vi "Control AlgorithmV3.vi"(6 "PID Gains":cluster{"P":dbl, "I":dbl, "D":dbl}, 7 "Init":bool, 8 "Motor to Control":u8, 9 "Manual Control":bool, 10 "Wheel Angles":dbl[](array[numeric]), 11 "JoystickIn":i32[](array[slide]) scale=-37626.0..37626.0) -> (2 "Target Angles":dbl[](array[numeric]), 3 "MotorsOut":u16[](array[slide]) scale=0.0..512.0)   [LabVIEW 2013, in "ProcessorHelperFunctions.lvlib"]
uses:
  ProcessorHelperFunctions.lvlib
panel:
  out "JoystickIn_DB":i32[](array[slide]) scale=-37626.0..37626.0
  out "y":dbl
  out "x":dbl
  out "Point":picture
  out "ReverseDir?4":bool
  out "ReverseDir?3":bool
  out "ReverseDir?2":bool
  out "ReverseDir?1":bool
  out "Radius1":dbl
  out "Radius2":dbl
  out "Radius3":dbl
  out "Radius4":dbl
  in  "RJoyMagGain":dbl=0.25
  in  "LJoyMagGain":dbl=1.0
  out "OldAngle4":dbl
  out "OldAngle3":dbl
  out "OldAngle2":dbl
  out "OldAngle1":dbl
  in  "Yw":dbl=15.5
  in  "Xw":dbl=21.5
  # "Xw is x distance between the\nwheels on the robot"
  # "------------------------------------ LOCAL VARIABLES ---------------------------------------"
  # "Yw is y distance between the\nwheels on the robot"
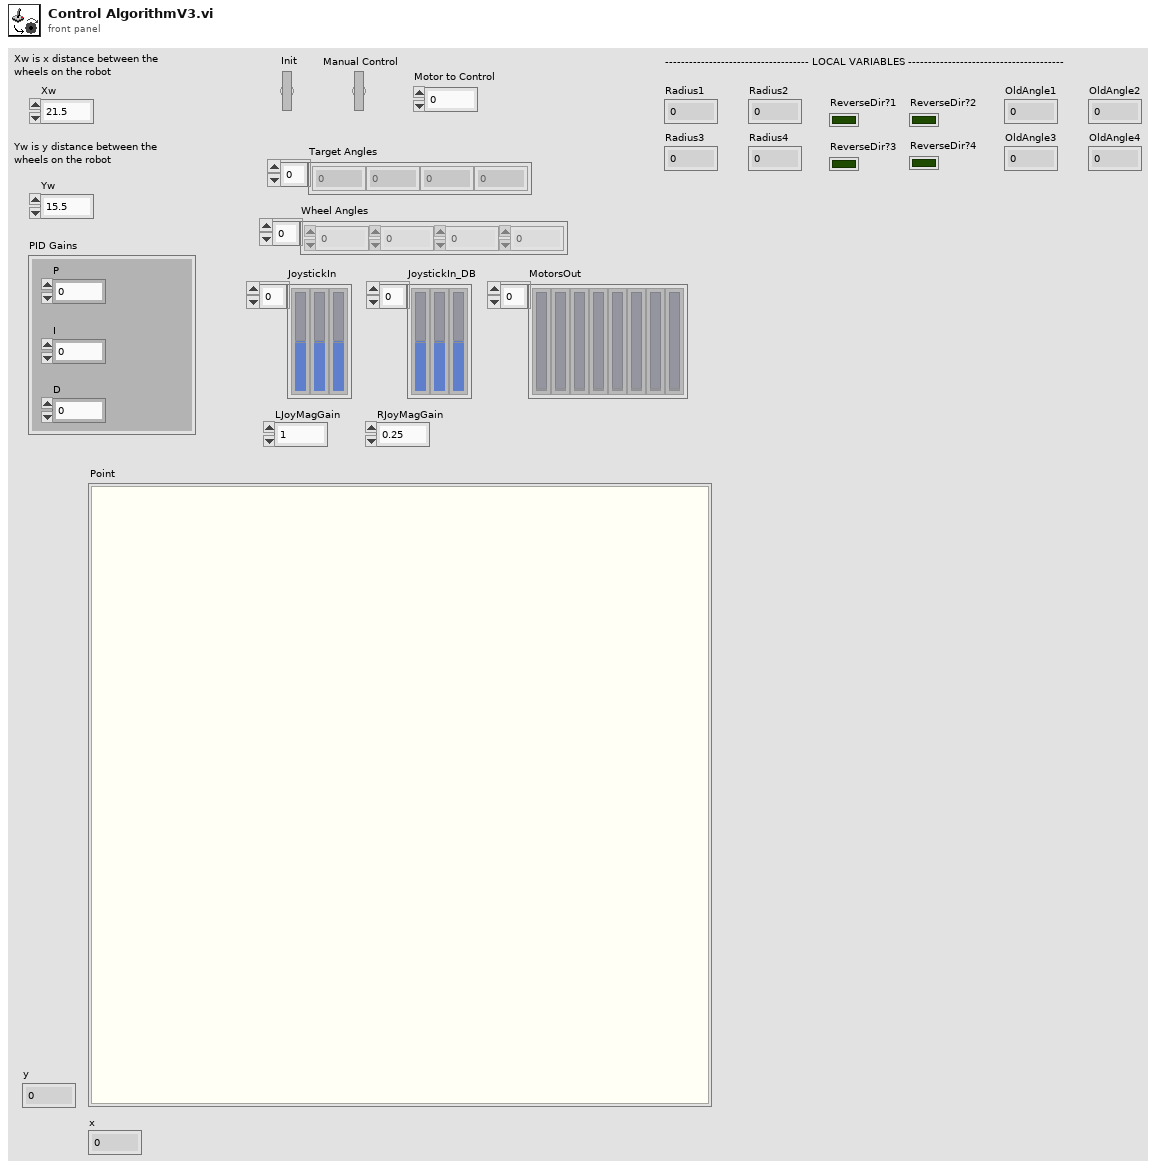
[diagram p1: front panel]
types:
  T1 = cluster{"Width":u16, "Style":enum32{"Solid", "Dash", "Dot", "DashDot", "DashDotDot"}}
  T2 = cluster{"JoystickOut[0]":i32, "JoystickOut[1]":i32, "JoystickOut[2]":i32, "JoystickOut[3]":i32, "JoystickOut[4]":i32, "JoystickOut[5]":i32, "JoystickOut[6]":i32, "JoystickOut[7]":i32, "JoystickOut[8]":i32}
  T3 = cluster{"Wheel Angles[0]":dbl, "Wheel Angles[1]":dbl, "Wheel Angles[2]":dbl, "Wheel Angles[3]":dbl, "Wheel Angles[4]":dbl, "Wheel Angles[5]":dbl, "Wheel Angles[6]":dbl, "Wheel Angles[7]":dbl, "Wheel Angles[8]":dbl}
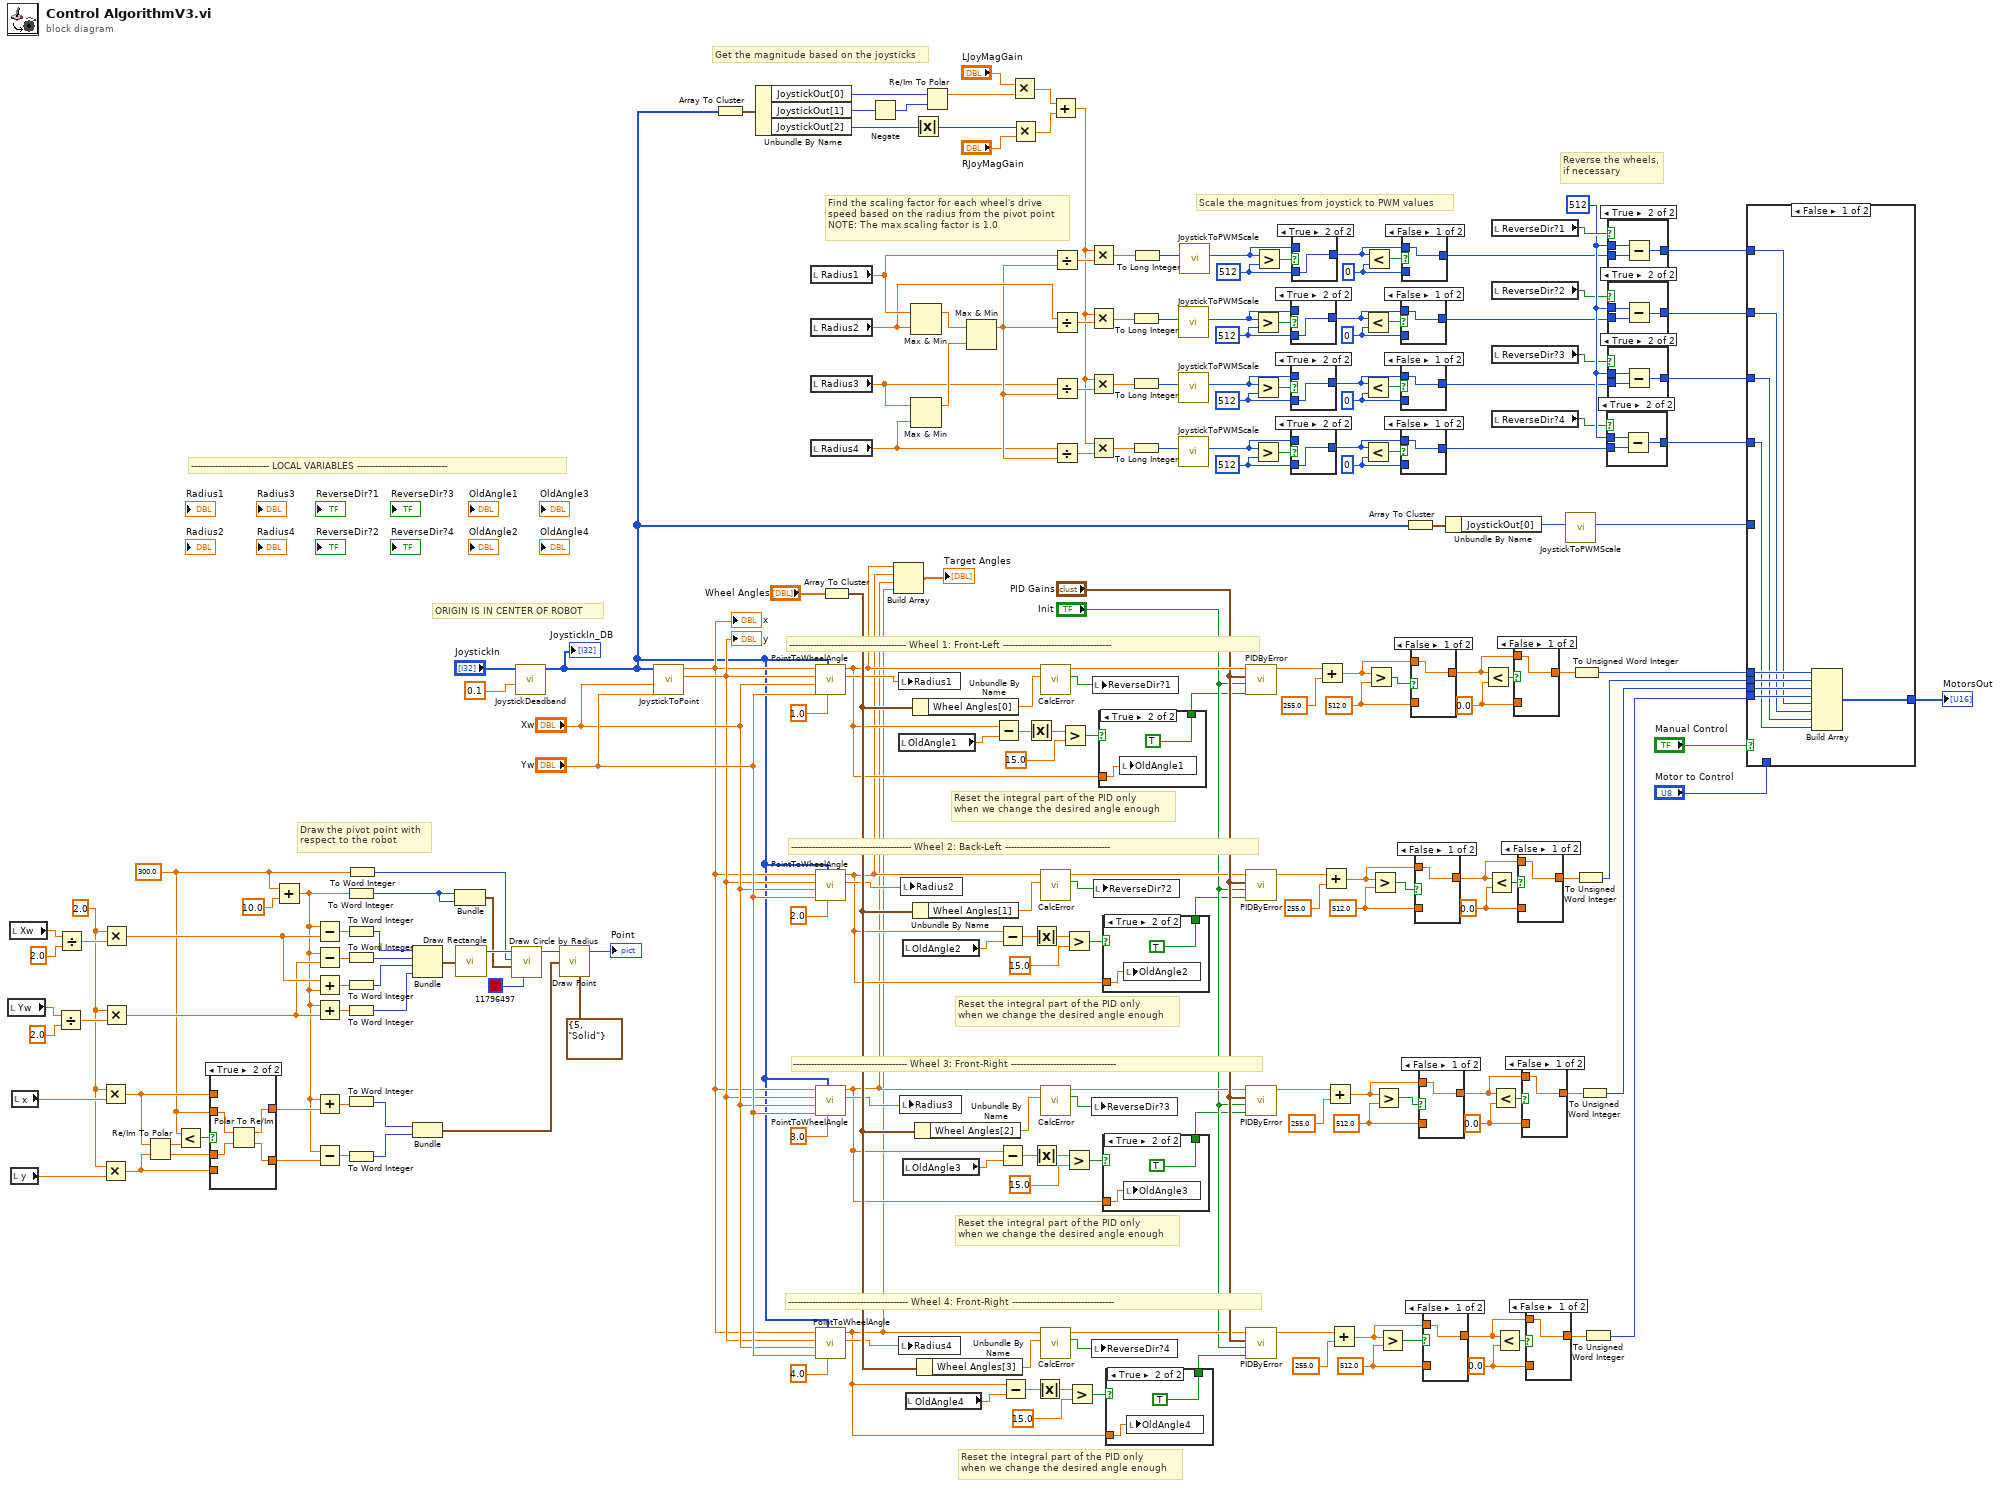
[diagram p0: block diagram]
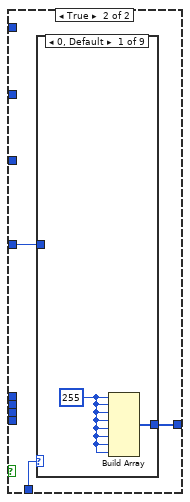
[diagram p15: hidden frame]
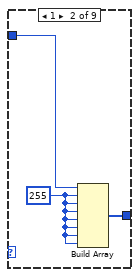
[diagram p16: hidden frame]
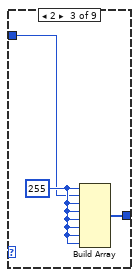
[diagram p17: hidden frame]
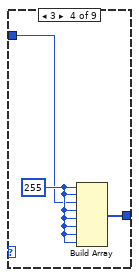
[diagram p18: hidden frame]
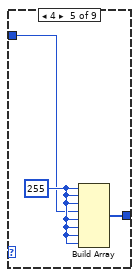
[diagram p19: hidden frame]
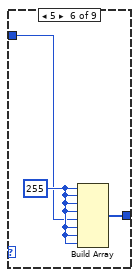
[diagram p20: hidden frame]
diagram:
  w7 = 0 ("y")
  w8 = 512 ("y")
  w18 = 0 ("y")
  w17 = 512 ("y")
  w25 = 0 ("y")
  w26 = 512 ("y")
  w41 = u16 512 ("x")
  w72 = 2.0 ("x")
  w53 = 300.0 ("x")
  w123 = 0 ("y")
  w122 = 512 ("y")
  w147 = 0.0 ("y")
  w145 = 512.0 ("y")
  w153 = 0.0 ("y")
  w155 = 512.0 ("y")
  w163 = 0.0 ("y")
  w161 = 512.0 ("y")
  w168 = 0.0 ("y")
  w170 = 512.0 ("y")
  # "Scale the magnitues from joystick to PWM values"
  # "Get the magnitude based on the joysticks"
  # "Reverse the wheels,\nif necessary"
  # "Draw the pivot point with\nrespect to the robot"
  # "Find the scaling factor for each wheel's drive\nspeed based on the radius from the pivot point\nNOTE: The max scaling factor is 1.0"
  # "Reset the integral part of the PID only\nwhen we change the desired angle enough"
  # "Reset the integral part of the PID only\nwhen we change the desired angle enough"
  # "Reset the integral part of the PID only\nwhen we change the desired angle enough"
  # "Reset the integral part of the PID only\nwhen we change the desired angle enough"
  # "-------------------------- LOCAL VARIABLES ------------------------------"
  # "---------------------------------------- Wheel 4: Front-Right ----------------------------------"
  # "-------------------------------------- Wheel 3: Front-Right -----------------------------------"
  # "---------------------------------------- Wheel 2: Back-Left -----------------------------------"
  # "--------------------------------------- Wheel 1: Front-Left ------------------------------------"
  # "ORIGIN IS IN CENTER OF ROBOT"
  n1 = local read "Yw"() -> (w97:dbl)
  n2 = local read "Xw"() -> (w100:dbl)
  n3 = local read "y"() -> (w73:dbl)
  n4 = local read "x"() -> (w80:dbl)
  n5 = Divide(x=w97, y=2.0) -> (x/y=w77:dbl)
  n6 = Divide(x=w100, y=2.0) -> (x/y=w78:dbl)
  n7 = Multiply(x=w72, y=w80) -> (x*y=w67:dbl)
  n8 = Multiply(x=w72, y=w73) -> (x*y=w66:dbl)
  n9 = Multiply(x=w72, y=w78) -> (x*y=w75:dbl)
  n10 = Multiply(x=w72, y=w77) -> (x*y=w74:dbl)
  n11 = Re/Im To Polar(2:w66, 3:w67) -> (0:w65:dbl, 1:w69:dbl)
  n12 = Less?(x=w53, y=w69) -> (x < y?=w68:bool)
  n13 = case shown="True" w68 {
    tunnel: w67 -> [w219 _]
    tunnel: w66 -> [w218 _]
    tunnel: w53 -> [_ w223]
    tunnel: w65 -> [_ w222]
    tunnel: [w219 w221] -> w63
    tunnel: [w218 w220] -> w64
    frame False {
    }
    frame True {
      n14 = Polar To Re/Im(2:w222, 3:w223) -> (0:w220:dbl, 1:w221:dbl)
    }
  }
  n15 = Add(x=w53, y=10.0) -> (x+y=w52:dbl)
  n16 = Subtract(x=w52, y=w75) -> (x-y=w58:dbl)
  n17 = Subtract(x=w52, y=w74) -> (x-y=w87:dbl)
  n18 = Add(x=w75, y=w52) -> (x+y=w86:dbl)
  n19 = Add(x=w52, y=w74) -> (x+y=w85:dbl)
  n20 = Add(x=w52, y=w63) -> (x+y=w62:dbl)
  n21 = Subtract(x=w52, y=w64) -> (x-y=w61:dbl)
  n22 = To Word Integer(number=w52) -> (16bit integer=w51:i16)
  n23 = To Word Integer(number=w58) -> (16bit integer=w88:i16)
  n24 = To Word Integer(number=w87) -> (16bit integer=w84:i16)
  n25 = To Word Integer(number=w86) -> (16bit integer=w83:i16)
  n26 = To Word Integer(number=w85) -> (16bit integer=w82:i16)
  n27 = To Word Integer(number=w62) -> (16bit integer=w96:i16)
  n28 = To Word Integer(number=w61) -> (16bit integer=w95:i16)
  n29 = To Word Integer(number=w53) -> (16bit integer=w55:i16)
  n30 = Bundle(w88, w84, w83, w82) -> (w81:cluster{i16, i16, i16, i16})  [unwired: 1 in]
  n31 = Bundle(w96, w95) -> (w94:cluster{i16, i16})  [unwired: 1 in]
  n32 = Bundle(w51, w51) -> (w57:cluster{i16, i16})  [unwired: 1 in]
  n33 = call <vilib>:"Draw Rectangle.vi"("rect"=w81) -> ("new picture"=w60:picture)  [unwired: 8 in]
  n34 = call <vilib>:"Draw Circle by Radius.vi"("color(black)"=u32 11796497, "pixel center"=w57, "radius"=w55, "picture"=w60) -> ("new picture"=w59:picture)  [unwired: 7 in]
  n35 = call "JoystickDeadband.vi"("DBPercent"=0.1, "JoystickIn"="JoystickIn") -> ("JoystickOut"=w2:i32[])  [unwired: 9 in]
  "JoystickIn_DB" <- w2
  n36 = call <vilib>:"Draw Point.vi"("picture"=w59, "point(x,y)"=w94, "pen"=T1 {"Width"=5, "Style"=enum."Solid"}) -> ("new picture"=→"Point":picture)  [unwired: 6 in]
  n37 = call "JoystickToPoint.vi"("Yw"="Yw", "Xw"="Xw", "JoystickIn"=w2) -> ("y"=w211:dbl, "x"=w210:dbl)  [unwired: 7 in]
  "x" <- w210
  "y" <- w211
  n38 = Array To Cluster(array=w2) -> (cluster=w134:T2)
  n39 = Unbundle By Name(w134) -> ("JoystickOut[0]"=w133:i32, "JoystickOut[1]"=w132:i32, "JoystickOut[2]"=w129:i32)
  n40 = local read "Radius1"() -> (w109:dbl)
  n41 = local read "Radius2"() -> (w108:dbl)
  n42 = local read "Radius3"() -> (w106:dbl)
  n43 = local read "Radius4"() -> (w105:dbl)
  n44 = call "PointToWheelAngle.vi"("Wheel Number"=1.0, "JoystickIn"=w2, "Yw"="Yw", "Xw"="Xw", "y"=w211, "x"=w210) -> ("Radius"=w119:dbl, "Desired Angle"=w50:dbl)  [unwired: 4 in]
  n45 = call "PointToWheelAngle.vi"("Wheel Number"=2.0, "JoystickIn"=w2, "Yw"="Yw", "Xw"="Xw", "y"=w211, "x"=w210) -> ("Radius"=w118:dbl, "Desired Angle"=w49:dbl)  [unwired: 4 in]
  n46 = call "PointToWheelAngle.vi"("Wheel Number"=3.0, "JoystickIn"=w2, "Yw"="Yw", "Xw"="Xw", "y"=w211, "x"=w210) -> ("Radius"=w117:dbl, "Desired Angle"=w48:dbl)  [unwired: 4 in]
  n47 = call "PointToWheelAngle.vi"("Wheel Number"=4.0, "JoystickIn"=w2, "Yw"="Yw", "Xw"="Xw", "y"=w211, "x"=w210) -> ("Radius"=w116:dbl, "Desired Angle"=w47:dbl)  [unwired: 4 in]
  n48 = Array To Cluster(array="Wheel Angles") -> (cluster=w208:T3)
  n49 = Negate(x=w132) -> (-x=w76:i32)
  n50 = Build Array(w50, w49, w48, w47) -> (→"Target Angles":dbl[])
  n51 = local write "Radius1"(w119) -> ()
  n52 = local read "OldAngle1"() -> (w198:dbl)
  n53 = local write "Radius4"(w116) -> ()
  n54 = local write "Radius3"(w117) -> ()
  n55 = local write "Radius2"(w118) -> ()
  n56 = local read "OldAngle2"() -> (w191:dbl)
  n57 = local read "OldAngle3"() -> (w186:dbl)
  n58 = local read "OldAngle4"() -> (w181:dbl)
  n59 = Max & Min(x=w109, y=w108) -> (max(x,y)=w111:dbl)  [unwired: 1 out]
  n60 = Max & Min(x=w106, y=w105) -> (max(x,y)=w110:dbl)  [unwired: 1 out]
  n61 = Absolute Value(x=w129) -> (abs(x)=w1:i32)
  n62 = Unbundle By Name(w208) -> ("Wheel Angles[0]"=w207:dbl)
  n63 = Unbundle By Name(w208) -> ("Wheel Angles[1]"=w206:dbl)
  n64 = Unbundle By Name(w208) -> ("Wheel Angles[2]"=w205:dbl)
  n65 = Unbundle By Name(w208) -> ("Wheel Angles[3]"=w204:dbl)
  n66 = Re/Im To Polar(2:w76, 3:w133) -> (1:w131:dbl)  [unwired: 1 out]
  n67 = Max & Min(x=w111, y=w110) -> (max(x,y)=w107:dbl)  [unwired: 1 out]
  n68 = Subtract(x=w50, y=w198) -> (x-y=w197:dbl)
  n69 = Subtract(x=w49, y=w191) -> (x-y=w190:dbl)
  n70 = Subtract(x=w48, y=w186) -> (x-y=w185:dbl)
  n71 = Subtract(x=w47, y=w181) -> (x-y=w180:dbl)
  n72 = Multiply(x="LJoyMagGain", y=w131) -> (x*y=w127:dbl)
  n73 = Multiply(x=w1, y="RJoyMagGain") -> (x*y=w126:dbl)
  n74 = Absolute Value(x=w197) -> (abs(x)=w196:dbl)
  n75 = Absolute Value(x=w190) -> (abs(x)=w189:dbl)
  n76 = Absolute Value(x=w185) -> (abs(x)=w184:dbl)
  n77 = Absolute Value(x=w180) -> (abs(x)=w179:dbl)
  n78 = call "CalcError.vi"("Actual Angle"=w207, "Desired Angle"=w50) -> ("ReverseDir?"=w115:bool, "Angle Error"=w203:dbl)  [unwired: 8 in]
  n79 = call "CalcError.vi"("Actual Angle"=w206, "Desired Angle"=w49) -> ("ReverseDir?"=w114:bool, "Angle Error"=w201:dbl)  [unwired: 8 in]
  n80 = call "CalcError.vi"("Actual Angle"=w205, "Desired Angle"=w48) -> ("ReverseDir?"=w113:bool, "Angle Error"=w200:dbl)  [unwired: 8 in]
  n81 = call "CalcError.vi"("Actual Angle"=w204, "Desired Angle"=w47) -> ("ReverseDir?"=w112:bool, "Angle Error"=w199:dbl)  [unwired: 8 in]
  n82 = Add(x=w127, y=w126) -> (x+y=w32:dbl)
  n83 = Divide(x=w109, y=w107) -> (x/y=w36:dbl)
  n84 = Divide(x=w108, y=w107) -> (x/y=w35:dbl)
  n85 = Divide(x=w106, y=w107) -> (x/y=w34:dbl)
  n86 = Divide(x=w105, y=w107) -> (x/y=w33:dbl)
  n87 = Greater?(x=w196, y=15.0) -> (0:w194:bool)
  n88 = Greater?(x=w189, y=15.0) -> (0:w187:bool)
  n89 = Greater?(x=w184, y=15.0) -> (0:w182:bool)
  n90 = Greater?(x=w179, y=15.0) -> (0:w177:bool)
  n91 = Multiply(x=w32, y=w36) -> (x*y=w31:dbl)
  n92 = Multiply(x=w32, y=w35) -> (x*y=w22:dbl)
  n93 = Multiply(x=w32, y=w34) -> (x*y=w13:dbl)
  n94 = Multiply(x=w32, y=w33) -> (x*y=w4:dbl)
  n95 = local write "ReverseDir?3"(w113) -> ()
  n96 = local write "ReverseDir?4"(w112) -> ()
  n97 = local write "ReverseDir?1"(w115) -> ()
  n98 = local write "ReverseDir?2"(w114) -> ()
  n99 = case shown="True" w194 {
    tunnel: w50 -> [_ w226]
    tunnel: [FALSE ("Reset1") TRUE ("Reset1")] -> w192
    frame False {
    }
    frame True {
      n100 = local write "OldAngle1"(w226) -> ()
    }
  }
  n101 = case shown="True" w187 {
    tunnel: w49 -> [_ w229]
    tunnel: [FALSE ("Reset1") TRUE ("Reset1")] -> w174
    frame False {
    }
    frame True {
      n102 = local write "OldAngle2"(w229) -> ()
    }
  }
  n103 = case shown="True" w182 {
    tunnel: w48 -> [_ w232]
    tunnel: [FALSE ("Reset1") TRUE ("Reset1")] -> w176
    frame False {
    }
    frame True {
      n104 = local write "OldAngle3"(w232) -> ()
    }
  }
  n105 = case shown="True" w177 {
    tunnel: w47 -> [_ w235]
    tunnel: [FALSE ("Reset1") TRUE ("Reset1")] -> w175
    frame False {
    }
    frame True {
      n106 = local write "OldAngle4"(w235) -> ()
    }
  }
  n107 = To Long Integer(number=w22) -> (32bit integer=w23:i32)
  n108 = To Long Integer(number=w13) -> (32bit integer=w20:i32)
  n109 = To Long Integer(number=w4) -> (32bit integer=w5:i32)
  n110 = To Long Integer(number=w31) -> (32bit integer=w125:i32)
  n111 = call "JoystickToPWMScale.vi"("Numeric"=w23) -> ("Numeric 2"=w28:u16)  [unwired: 10 in]
  n112 = call "JoystickToPWMScale.vi"("Numeric"=w20) -> ("Numeric 2"=w15:u16)  [unwired: 10 in]
  n113 = call "JoystickToPWMScale.vi"("Numeric"=w5) -> ("Numeric 2"=w10:u16)  [unwired: 10 in]
  n114 = call "JoystickToPWMScale.vi"("Numeric"=w125) -> ("Numeric 2"=w120:u16)  [unwired: 10 in]
  n115 = call "PIDByError.vi"("Error"=w203, "PID Gains"="PID Gains", "Init"="Init", "Reset"=w192) -> ("Control"=w173:dbl)  [unwired: 6 in]
  n116 = call "PIDByError.vi"("Error"=w201, "PID Gains"="PID Gains", "Init"="Init", "Reset"=w174) -> ("Control"=w158:dbl)  [unwired: 6 in]
  n117 = call "PIDByError.vi"("Error"=w200, "PID Gains"="PID Gains", "Init"="Init", "Reset"=w176) -> ("Control"=w150:dbl)  [unwired: 6 in]
  n118 = call "PIDByError.vi"("Error"=w199, "PID Gains"="PID Gains", "Init"="Init", "Reset"=w175) -> ("Control"=w142:dbl)  [unwired: 6 in]
  n119 = Greater?(x=w28, y=w26) -> (0:w27:bool)
  n120 = Greater?(x=w15, y=w17) -> (0:w16:bool)
  n121 = Greater?(x=w10, y=w8) -> (0:w9:bool)
  n122 = Greater?(x=w120, y=w122) -> (0:w121:bool)
  n123 = case shown="True" w27 {
    tunnel: w26 -> [_ w237]
    tunnel: w28 -> [w236 _]
    tunnel: [w236 w237] -> w24
    frame False {
    }
    frame True {
    }
  }
  n124 = case shown="True" w16 {
    tunnel: w17 -> [_ w239]
    tunnel: w15 -> [w238 _]
    tunnel: [w238 w239] -> w19
    frame False {
    }
    frame True {
    }
  }
  n125 = case shown="True" w9 {
    tunnel: w8 -> [_ w241]
    tunnel: w10 -> [w240 _]
    tunnel: [w240 w241] -> w6
    frame False {
    }
    frame True {
    }
  }
  n126 = case shown="True" w121 {
    tunnel: w122 -> [_ w243]
    tunnel: w120 -> [w242 _]
    tunnel: [w242 w243] -> w124
    frame False {
    }
    frame True {
    }
  }
  n127 = Add(x=w173, y=255.0) -> (x+y=w169:dbl)
  n128 = Add(x=w158, y=255.0) -> (x+y=w162:dbl)
  n129 = Add(x=w150, y=255.0) -> (x+y=w154:dbl)
  n130 = Add(x=w142, y=255.0) -> (x+y=w146:dbl)
  n131 = Less?(x=w24, y=w25) -> (x < y?=w29:bool)
  n132 = Less?(x=w19, y=w18) -> (x < y?=w14:bool)
  n133 = Less?(x=w6, y=w7) -> (x < y?=w11:bool)
  n134 = Less?(x=w124, y=w123) -> (x < y?=w89:bool)
  n135 = Greater?(x=w169, y=w170) -> (0:w171:bool)
  n136 = Greater?(x=w162, y=w161) -> (0:w160:bool)
  n137 = Greater?(x=w154, y=w155) -> (0:w156:bool)
  n138 = Greater?(x=w146, y=w145) -> (0:w144:bool)
  n139 = case shown="False" w29 {
    tunnel: w25 -> [_ w245]
    tunnel: w24 -> [w244 _]
    tunnel: [w244 w245] -> w21
    frame False {
    }
    frame True {
    }
  }
  n140 = case shown="False" w14 {
    tunnel: w18 -> [_ w247]
    tunnel: w19 -> [w246 _]
    tunnel: [w246 w247] -> w12
    frame False {
    }
    frame True {
    }
  }
  n141 = case shown="False" w11 {
    tunnel: w7 -> [_ w249]
    tunnel: w6 -> [w248 _]
    tunnel: [w248 w249] -> w3
    frame False {
    }
    frame True {
    }
  }
  n142 = case shown="False" w89 {
    tunnel: w123 -> [_ w251]
    tunnel: w124 -> [w250 _]
    tunnel: [w250 w251] -> w30
    frame False {
    }
    frame True {
    }
  }
  n143 = Array To Cluster(array=w2) -> (cluster=w104:T2)
  n144 = case shown="False" w171 {
    tunnel: w170 -> [_ w253]
    tunnel: w169 -> [w252 _]
    tunnel: [w252 w253] -> w167
    frame False {
    }
    frame True {
    }
  }
  n145 = case shown="False" w160 {
    tunnel: w161 -> [_ w255]
    tunnel: w162 -> [w254 _]
    tunnel: [w254 w255] -> w164
    frame False {
    }
    frame True {
    }
  }
  n146 = case shown="False" w156 {
    tunnel: w155 -> [_ w257]
    tunnel: w154 -> [w256 _]
    tunnel: [w256 w257] -> w152
    frame False {
    }
    frame True {
    }
  }
  n147 = case shown="False" w144 {
    tunnel: w145 -> [_ w259]
    tunnel: w146 -> [w258 _]
    tunnel: [w258 w259] -> w148
    frame False {
    }
    frame True {
    }
  }
  n148 = Unbundle By Name(w104) -> ("JoystickOut[0]"=w103:i32)
  n149 = Less?(x=w167, y=w168) -> (x < y?=w90:bool)
  n150 = Less?(x=w164, y=w163) -> (x < y?=w91:bool)
  n151 = Less?(x=w152, y=w153) -> (x < y?=w92:bool)
  n152 = local read "ReverseDir?1"() -> (w45:bool)
  n153 = local read "ReverseDir?2"() -> (w39:bool)
  n154 = local read "ReverseDir?3"() -> (w38:bool)
  n155 = local read "ReverseDir?4"() -> (w37:bool)
  n156 = Less?(x=w148, y=w147) -> (x < y?=w93:bool)
  n157 = case shown="False" w90 {
    tunnel: w168 -> [_ w261]
    tunnel: w167 -> [w260 _]
    tunnel: [w260 w261] -> w166
    frame False {
    }
    frame True {
    }
  }
  n158 = case shown="False" w91 {
    tunnel: w163 -> [_ w263]
    tunnel: w164 -> [w262 _]
    tunnel: [w262 w263] -> w165
    frame False {
    }
    frame True {
    }
  }
  n159 = case shown="False" w92 {
    tunnel: w153 -> [_ w265]
    tunnel: w152 -> [w264 _]
    tunnel: [w264 w265] -> w151
    frame False {
    }
    frame True {
    }
  }
  n160 = case shown="False" w93 {
    tunnel: w147 -> [_ w267]
    tunnel: w148 -> [w266 _]
    tunnel: [w266 w267] -> w149
    frame False {
    }
    frame True {
    }
  }
  n161 = call "JoystickToPWMScale.vi"("Numeric"=w103) -> ("Numeric 2"=w102:u16)  [unwired: 10 in]
  n162 = To Unsigned Word Integer(number=w166) -> (unsigned 16bit integer=w141:u16)
  n163 = To Unsigned Word Integer(number=w165) -> (unsigned 16bit integer=w140:u16)
  n164 = To Unsigned Word Integer(number=w151) -> (unsigned 16bit integer=w139:u16)
  n165 = To Unsigned Word Integer(number=w149) -> (unsigned 16bit integer=w138:u16)
  n166 = case shown="True" w37 {
    tunnel: w3 -> [w268 w271]
    tunnel: w41 -> [_ w270]
    tunnel: [w268 w269] -> w40
    frame False {
    }
    frame True {
      n167 = Subtract(x=w270, y=w271) -> (x-y=w269:i32)
    }
  }
  n168 = case shown="True" w45 {
    tunnel: w30 -> [w272 w275]
    tunnel: w41 -> [_ w274]
    tunnel: [w272 w273] -> w44
    frame False {
    }
    frame True {
      n169 = Subtract(x=w274, y=w275) -> (x-y=w273:i32)
    }
  }
  n170 = case shown="True" w39 {
    tunnel: w21 -> [w276 w279]
    tunnel: w41 -> [_ w278]
    tunnel: [w276 w277] -> w42
    frame False {
    }
    frame True {
      n171 = Subtract(x=w278, y=w279) -> (x-y=w277:i32)
    }
  }
  n172 = case shown="True" w38 {
    tunnel: w12 -> [w280 w283]
    tunnel: w41 -> [_ w282]
    tunnel: [w280 w281] -> w43
    frame False {
    }
    frame True {
      n173 = Subtract(x=w282, y=w283) -> (x-y=w281:i32)
    }
  }
  n174 = case shown="False" "Manual Control" {
    tunnel: w141 -> [w292 _]
    tunnel: w140 -> [w291 _]
    tunnel: w139 -> [w290 _]
    tunnel: w138 -> [w289 _]
    tunnel: [w288 w293] -> w137
    tunnel: "Motor to Control" -> [_ w295]
    tunnel: w44 -> [w287 _]
    tunnel: w42 -> [w286 _]
    tunnel: w43 -> [w284 _]
    tunnel: w40 -> [w285 _]
    tunnel: w102 -> [_ w294]
    frame False {
      n175 = Build Array(w292, w291, w290, w289, w287, w286, w284, w285) -> (w288:i32[])
    }
    frame True {
      n176 = case shown="0, Default" w295 {
        tunnel: w294 -> [_ w298 w301 w304 w307 w310 w313 w316 w319]
        tunnel: [w297 w299 w302 w305 w308 w311 w314 w317 w320] -> w293
        frame 0, Default {
          w296 = 255
          n177 = Build Array(w296, w296, w296, w296, w296, w296, w296, w296) -> (w297:i32[])
        }
        frame 1 {
          w300 = 255
          n178 = Build Array(w298, w300, w300, w300, w300, w300, w300, w300) -> (w299:i32[])
        }
        frame 2 {
          w303 = 255
          n179 = Build Array(w303, w301, w303, w303, w303, w303, w303, w303) -> (w302:i32[])
        }
        frame 3 {
          w306 = 255
          n180 = Build Array(w306, w306, w304, w306, w306, w306, w306, w306) -> (w305:i32[])
        }
        frame 4 {
          w309 = 255
          n181 = Build Array(w309, w309, w309, w307, w309, w309, w309, w309) -> (w308:i32[])
        }
        frame 5 {
          w312 = 255
          n182 = Build Array(w312, w312, w312, w312, w310, w312, w312, w312) -> (w311:i32[])
        }
        frame 6 {
          w315 = 255
          n183 = Build Array(w315, w315, w315, w315, w315, w313, w315, w315) -> (w314:i32[])
        }
        frame 7 {
          w318 = 255
          n184 = Build Array(w318, w318, w318, w318, w318, w318, w316, w318) -> (w317:i32[])
        }
        frame 8 {
          w321 = 255
          n185 = Build Array(w321, w321, w321, w321, w321, w321, w321, w319) -> (w320:i32[])
        }
      }
    }
  }
  "MotorsOut" <- w137
